vi "Set Uim MCFG wrapper.vi"(7 "bAckEna":i32, 8 "error in (no error)":errorcluster caption="错误输入（无错误）", 9 "UIM_MCFG_INFO_OBJ In":T1, 10 "dwCanNodeId":u32, 11 "dwDevIndex":u32) -> (0 "error out":errorcluster caption="错误输出", 1 "UIM_MCFG_INFO_OBJ Out":T1, 3 "function return":u32)   [LabVIEW 2016, in "UISimCanFunc_wrapper.lvlib"]
doc: "_declspec (dllexport) DWORD SetUimMCFG_wrapper(DWORD dwDevIndex, DWORD dwCanNodeId,\n P_DUMMY_UIM_MCFG_INFO_OBJ pDummyMCFGInfoIn, BOOL bAckEna, P_DUMMY_UIM_MCFG_INFO_OBJ pDummyMCFGInfoOut);"
uses:
  <userlib>/UISimCanFunc_wrapper/UISimCanFunc_wrapper.lvlib
  <userlib>/UISimCanFunc_wrapper/ctl/UIM_MCFG_INFO_OBJ.ctl
  <userlib>/UISimCanFunc_wrapper/UISimCanFunc_wrapper.dll
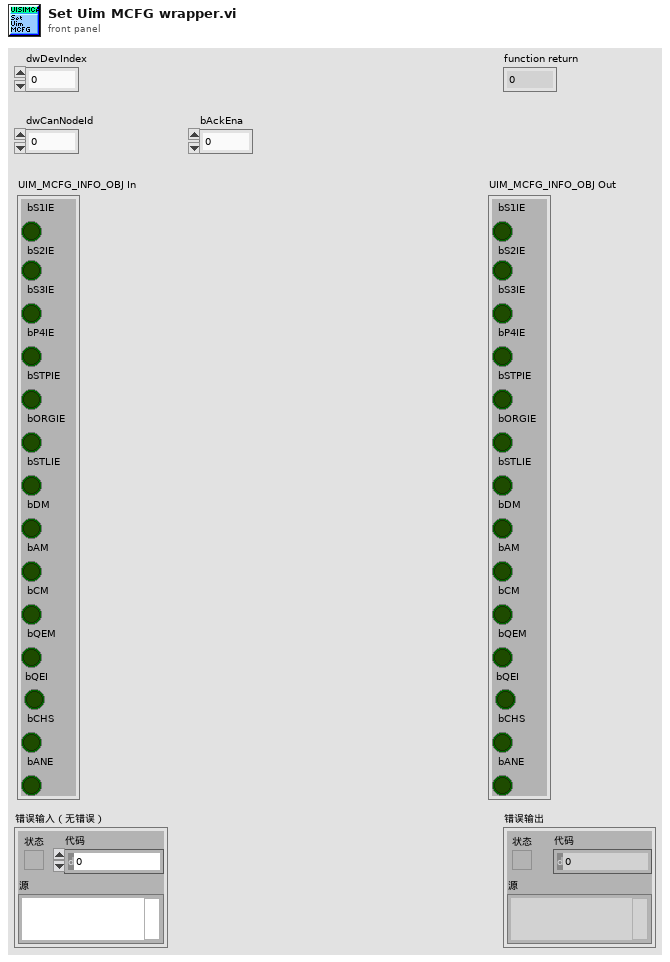
[diagram p1: front panel]
types:
  T1 = typedef "UISimCanFunc_wrapper.lvlib/UIM_MCFG_INFO_OBJ.ctl" = cluster{" bS1IE":bool, " bS2IE":bool, " bS3IE":bool, " bP4IE":bool, " bSTPIE":bool, " bORGIE":bool, " bSTLIE":bool, " bDM":bool, " bAM":bool, " bCM":bool, " bQEM":bool, " bQEI        ":bool, " bCHS":bool, " bANE":bool}
  T2 = cluster{"bS1IE":i32, "bS2IE":i32, "bS3IE":i32, "bP4IE":i32, "bSTPIE":i32, "bORGIE":i32, "bSTLIE":i32, "bDM":i32, "bAM":i32, "bCM":i32, "bQEM":i32, "bQEI":i32, "bCHS":i32, "bANE":i32}
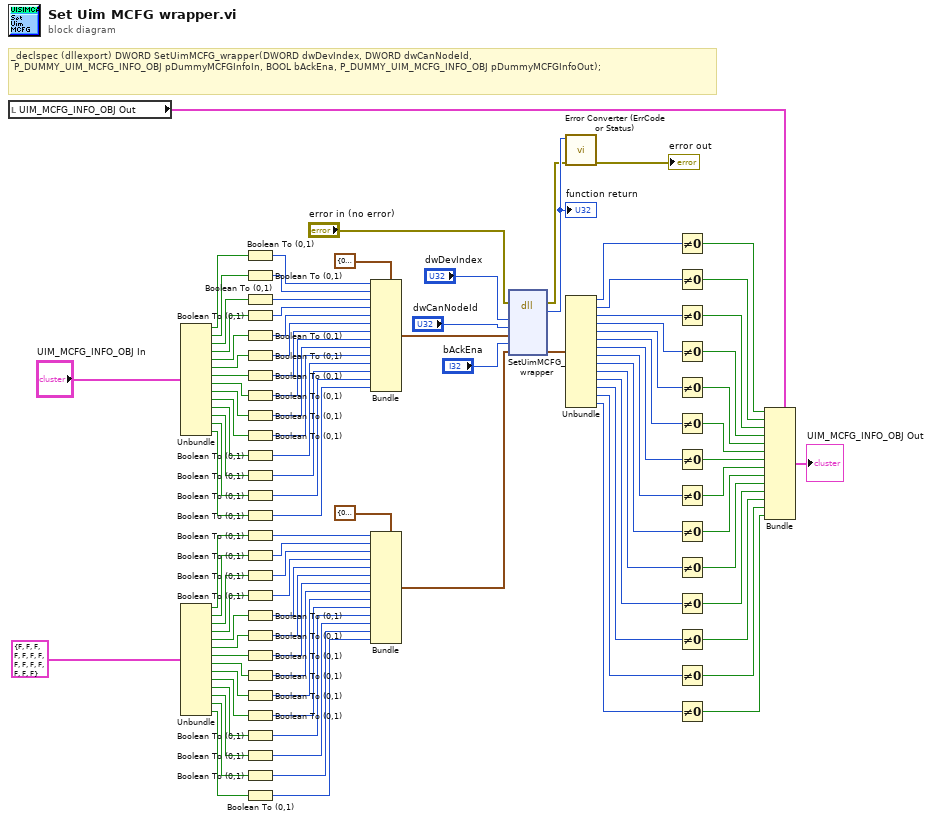
[diagram p0: block diagram]
diagram:
  # "_declspec (dllexport) DWORD SetUimMCFG_wrapper(DWORD dwDevIndex, DWORD dwCanNodeId,\n\tP_DUMMY_UIM_MCFG_INFO_OBJ pDummyMCFGInfoIn, BOOL bAckEna, P_DUMMY_UIM_MCFG_INFO_OBJ pDummyMCFGInfoOut);"
  n1 = local read "UIM_MCFG_INFO_OBJ Out"() -> (w93:T1)
  n2 = Unbundle("UIM_MCFG_INFO_OBJ In") -> ("bS1IE"=w60:bool, "bS2IE"=w59:bool, "bS3IE"=w58:bool, "bP4IE"=w57:bool, "bSTPIE"=w56:bool, "bORGIE"=w55:bool, "bSTLIE"=w54:bool, "bDM"=w53:bool, "bAM"=w52:bool, "bCM"=w51:bool, "bQEM"=w50:bool, "bQEI"=w49:bool, "bCHS"=w48:bool, "bANE"=w47:bool)
  n3 = Unbundle(T1 {" bS1IE"=FALSE, " bS2IE"=FALSE, " bS3IE"=FALSE, " bP4IE"=FALSE, " bSTPIE"=FALSE, " bORGIE"=FALSE, " bSTLIE"=FALSE, " bDM"=FALSE, " bAM"=FALSE, " bCM"=FALSE, " bQEM"=FALSE, " bQEI        "=FALSE, " bCHS"=FALSE, " bANE"=FALSE} ("UIM_MCFG_INFO_OBJ")) -> ("bS1IE"=w29:bool, "bS2IE"=w28:bool, "bS3IE"=w27:bool, "bP4IE"=w26:bool, "bSTPIE"=w25:bool, "bORGIE"=w24:bool, "bSTLIE"=w23:bool, "bDM"=w22:bool, "bAM"=w21:bool, "bCM"=w20:bool, "bQEM"=w19:bool, "bQEI"=w18:bool, "bCHS"=w17:bool, "bANE"=w16:bool)
  n4 = Boolean To (0,1)(Boolean=w60) -> (0, 1=w46:i16)
  n5 = Boolean To (0,1)(Boolean=w59) -> (0, 1=w45:i16)
  n6 = Boolean To (0,1)(Boolean=w58) -> (0, 1=w44:i16)
  n7 = Boolean To (0,1)(Boolean=w57) -> (0, 1=w43:i16)
  n8 = Boolean To (0,1)(Boolean=w56) -> (0, 1=w42:i16)
  n9 = Boolean To (0,1)(Boolean=w55) -> (0, 1=w41:i16)
  n10 = Boolean To (0,1)(Boolean=w54) -> (0, 1=w40:i16)
  n11 = Boolean To (0,1)(Boolean=w53) -> (0, 1=w39:i16)
  n12 = Boolean To (0,1)(Boolean=w52) -> (0, 1=w38:i16)
  n13 = Boolean To (0,1)(Boolean=w51) -> (0, 1=w37:i16)
  n14 = Boolean To (0,1)(Boolean=w50) -> (0, 1=w36:i16)
  n15 = Boolean To (0,1)(Boolean=w49) -> (0, 1=w35:i16)
  n16 = Boolean To (0,1)(Boolean=w48) -> (0, 1=w34:i16)
  n17 = Boolean To (0,1)(Boolean=w47) -> (0, 1=w33:i16)
  n18 = Boolean To (0,1)(Boolean=w29) -> (0, 1=w15:i16)
  n19 = Boolean To (0,1)(Boolean=w28) -> (0, 1=w14:i16)
  n20 = Boolean To (0,1)(Boolean=w27) -> (0, 1=w13:i16)
  n21 = Boolean To (0,1)(Boolean=w26) -> (0, 1=w12:i16)
  n22 = Boolean To (0,1)(Boolean=w25) -> (0, 1=w11:i16)
  n23 = Boolean To (0,1)(Boolean=w24) -> (0, 1=w10:i16)
  n24 = Boolean To (0,1)(Boolean=w23) -> (0, 1=w9:i16)
  n25 = Boolean To (0,1)(Boolean=w22) -> (0, 1=w8:i16)
  n26 = Boolean To (0,1)(Boolean=w21) -> (0, 1=w7:i16)
  n27 = Boolean To (0,1)(Boolean=w20) -> (0, 1=w6:i16)
  n28 = Boolean To (0,1)(Boolean=w19) -> (0, 1=w5:i16)
  n29 = Boolean To (0,1)(Boolean=w18) -> (0, 1=w4:i16)
  n30 = Boolean To (0,1)(Boolean=w17) -> (0, 1=w3:i16)
  n31 = Boolean To (0,1)(Boolean=w16) -> (0, 1=w2:i16)
  n32 = Bundle(cluster=T2 {"bS1IE"=0, "bS2IE"=0, "bS3IE"=0, "bP4IE"=0, "bSTPIE"=0, "bORGIE"=0, "bSTLIE"=0, "bDM"=0, "bAM"=0, "bCM"=0, "bQEM"=0, "bQEI"=0, "bCHS"=0, "bANE"=0} ("pDummyMCFGInfo"), "bS1IE"=w46, "bS2IE"=w45, "bS3IE"=w44, "bP4IE"=w43, "bSTPIE"=w42, "bORGIE"=w41, "bSTLIE"=w40, "bDM"=w39, "bAM"=w38, "bCM"=w37, "bQEM"=w36, "bQEI"=w35, "bCHS"=w34, "bANE"=w33) -> (w32:T2)
  n33 = Bundle(cluster=T2 {"bS1IE"=0, "bS2IE"=0, "bS3IE"=0, "bP4IE"=0, "bSTPIE"=0, "bORGIE"=0, "bSTLIE"=0, "bDM"=0, "bAM"=0, "bCM"=0, "bQEM"=0, "bQEI"=0, "bCHS"=0, "bANE"=0} ("pDummyMCFGInfo"), "bS1IE"=w15, "bS2IE"=w14, "bS3IE"=w13, "bP4IE"=w12, "bSTPIE"=w11, "bORGIE"=w10, "bSTLIE"=w9, "bDM"=w8, "bAM"=w7, "bCM"=w6, "bQEM"=w5, "bQEI"=w4, "bCHS"=w3, "bANE"=w2) -> (w1:T2)
  n34 = dll-call lib="C:/Program Files (x86)/National Instruments/LabVIEW 2016/user.lib/UISimCanFunc_wrapper/UISimCanFunc_wrapper.*" fn="SetUimMCFG_wrapper"(error in="error in (no error)", "dwDevIndex"="dwDevIndex", "dwCanNodeId"="dwCanNodeId", "pDummyMCFGInfoIn"=w32, "bAckEna"="bAckEna", "pDummyMCFGInfoOut"=w1) -> (error out=w95:errorcluster, w100:u32, "pDummyMCFGInfoOut"=w91:T2)  [unwired: 6 in, 1 out]
  "function return" <- w100
  n35 = call <userlib>:"Error Converter (ErrCode or Status).vi"("error in (no error)"=w95, "error code"=w100) -> ("error out"=→"error out":errorcluster)  [unwired: 9 in]
  n36 = Unbundle(w91) -> ("bS1IE"=w90:i32, "bS2IE"=w88:i32, "bS3IE"=w86:i32, "bP4IE"=w84:i32, "bSTPIE"=w82:i32, "bORGIE"=w80:i32, "bSTLIE"=w78:i32, "bDM"=w76:i32, "bAM"=w74:i32, "bCM"=w72:i32, "bQEM"=w70:i32, "bQEI"=w68:i32, "bCHS"=w66:i32, "bANE"=w64:i32)
  n37 = Not Equal To 0?(x=w90) -> (x != 0?=w89:bool)
  n38 = Not Equal To 0?(x=w88) -> (x != 0?=w87:bool)
  n39 = Not Equal To 0?(x=w86) -> (x != 0?=w85:bool)
  n40 = Not Equal To 0?(x=w84) -> (x != 0?=w83:bool)
  n41 = Not Equal To 0?(x=w82) -> (x != 0?=w81:bool)
  n42 = Not Equal To 0?(x=w80) -> (x != 0?=w79:bool)
  n43 = Not Equal To 0?(x=w78) -> (x != 0?=w77:bool)
  n44 = Not Equal To 0?(x=w76) -> (x != 0?=w75:bool)
  n45 = Not Equal To 0?(x=w74) -> (x != 0?=w73:bool)
  n46 = Not Equal To 0?(x=w72) -> (x != 0?=w71:bool)
  n47 = Not Equal To 0?(x=w70) -> (x != 0?=w69:bool)
  n48 = Not Equal To 0?(x=w68) -> (x != 0?=w67:bool)
  n49 = Not Equal To 0?(x=w66) -> (x != 0?=w65:bool)
  n50 = Not Equal To 0?(x=w64) -> (x != 0?=w63:bool)
  n51 = Bundle(cluster=w93, "bS1IE"=w89, "bS2IE"=w87, "bS3IE"=w85, "bP4IE"=w83, "bSTPIE"=w81, "bORGIE"=w79, "bSTLIE"=w77, "bDM"=w75, "bAM"=w73, "bCM"=w71, "bQEM"=w69, "bQEI"=w67, "bCHS"=w65, "bANE"=w63) -> (→"UIM_MCFG_INFO_OBJ Out":T1)
